vi "CRYAna Time.vi"(0 "Time Option":bool[](array[boolean]), 1 "Graph Info":T7={"Fs"=44100.0, "Channel Name"="Left", "Make Fundamental curve?"=FALSE}, 2 "TSR Info":T6 {"Impulse Resp Y" format="%.2f"; "Impulse Resp X" format="%.2f"}, 3 "Additive Info":T3, 5 "Stimulus":dbl[](array[numeric]), 7 "Input Info":T9, 9 "Response":dbl[](array[numeric]), 11 "Unit Info":T4={"Y unit In"="dB", "dB ref In"=1.0, "Y unit Out"="dB", "dB ref Out"=1.0, "Y unit Curve"="dB", "dB ref Curve"=1.0, "Y data  Curve"=0, "Y data Time"=0}, 12 "Algorithm":u16, 13 "Result Waveform":T8, 14 "EQ information":T2={"Stimulus EQ Curve"={"Name"="", "Curve"=[], "X data"=1, "Y data"=1, "Z data"=1, "X axis"=0, "Y axis"=1, "Z axis"=1, "X unit"="Hz", "Y unit"="", "Z unit"="deg.", "X dB ref"=1.0, "Y dB ref"=1.0, "Z dB ref"=1.0, "single val"=FALSE, "protected"=FALSE, "display X"=TRUE, "display Y"=TRUE, "display Z"=TRUE, "Test Info"="", "Step No."=0, "Plot Settings"={"Color"=0, "Interpolation"=0, "Point Style"=0, "Line Style"=0, "Point Color"=0, "Line Width"=0, "Bar Plot Style"=0, "Fill To"=0}, "AutoProtect"=FALSE}, "EQ"=FALSE, "EQ Rate"=0.0} {"EQ Rate" format="%.2f"; "Stimulus EQ Curve"."Z data" items=["dB", "Lin"]; "Stimulus EQ Curve"."X data" items=["dB", "Lin"]; "Stimulus EQ Curve"."Y data" items=["dB", "Lin"]; "Stimulus EQ Curve"."Z dB ref" format="%.1f"; "Stimulus EQ Curve"."Z axis" items=["Log", "Lin"]; "Stimulus EQ Curve"."X dB ref" format="%.1f"; "Stimulus EQ Curve"."X axis" items=["Log", "Lin"]; "Stimulus EQ Curve"."Y axis" items=["Log", "Lin"]; "Stimulus EQ Curve"."Y dB ref" format="%.1f"; "Stimulus EQ Curve"."Curve"."z" format="%.2f"; "Stimulus EQ Curve"."Curve"."y" format="%.2f"; "Stimulus EQ Curve"."Curve"."x" format="%.2f"}) -> (4 "Wave out":T5[](array[typedef]) {"Y dB ref" format="%.1f"; "Y axis" items=["Log", "Lin"]; "Y data" items=["dB", "Lin"]; "X data" items=["dB", "Lin"]})   [LabVIEW 2013]
uses:
  Typedef Control/CRYWaveform Cluster.ctl
  Typedef Control/CRYUnit Info Cluster.ctl
  Typedef Control/CRYData Cluster.ctl
  Typedef Control/CRYStimulus Test Infor Cluster.ctl
panel:
  in  "Waveform Cluster Out":T5={"Waveform"={"X0"=0.0, "dX"=0.0, "Y"=[]}, "X data"=1, "Y data"=0, "Y axis"=0, "X unit"="s", "Y unit"="", "Y dB ref"=1.0, "display Y"=TRUE, "display X"=FALSE, "Overload?"=FALSE, "Test Info"="", "Step No."=0, "Name"="", "protected"=FALSE, "Sqc history"=[], "Signal Channel ID"=0, "Plot Settings"={"Color"=0, "Interpolation"=0, "Point Style"=0, "Line Style"=0, "Point Color"=0, "Line Width"=0, "Bar Plot Style"=0, "Fill To"=0}, "AutoProtect"=FALSE} {"Y dB ref" format="%.1f"; "Y axis" items=["Log", "Lin"]; "Y data" items=["dB", "Lin"]; "X data" items=["dB", "Lin"]}
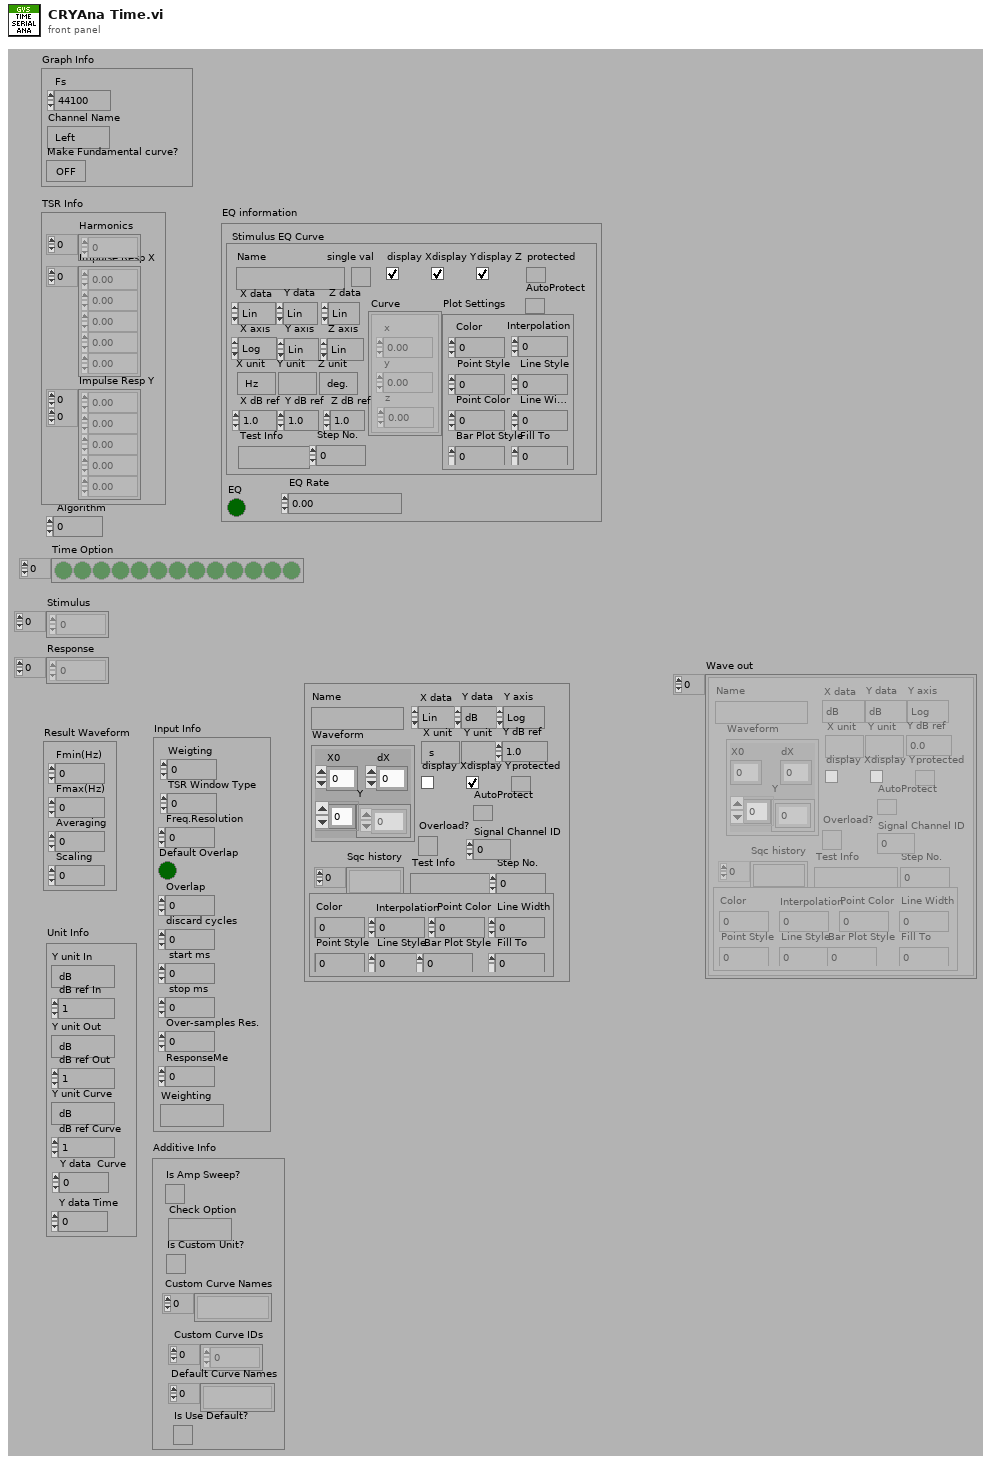
[diagram p1: front panel]
types:
  T1 = typedef "CRYData Cluster.ctl" = cluster{"Name":string, "Curve":cluster{"x":dbl, "y":dbl, "z":dbl}[], "X data":u16, "Y data":u16, "Z data":u16, "X axis":u16, "Y axis":u16, "Z axis":u16, "X unit":string, "Y unit":string, "Z unit":string, "X dB ref":dbl, "Y dB ref":dbl, "Z dB ref":dbl, "single val":bool, "protected":bool, "display X":bool, "display Y":bool, "display Z":bool, "Test Info":string, "Step No.":i32, "Plot Settings":cluster{"Color":u32, "Interpolation":u8, "Point Style":u8, "Line Style":u8, "Point Color":u32, "Line Width":u8, "Bar Plot Style":u8, "Fill To":i16}, "AutoProtect":bool}
  T2 = cluster{"Stimulus EQ Curve":T1, "EQ":bool, "EQ Rate":dbl}
  T3 = cluster{"Is Amp Sweep?":bool, "Check Option":string, "Is Custom Unit?":bool, "Custom Curve Names":string[], "Custom Curve IDs":i32[], "Default Curve Names":string[], "Is Use Default?":bool}
  T4 = typedef "CRYUnit Info Cluster.ctl" = cluster{"Y unit In":string, "dB ref In":dbl, "Y unit Out":string, "dB ref Out":dbl, "Y unit Curve":string, "dB ref Curve":dbl, "Y data  Curve":u16, "Y data Time":u16}
  T5 = typedef "CRYWaveform Cluster.ctl" = cluster{"Waveform":cluster{"X0":dbl, "dX":dbl, "Y":sgl[]}, "X data":u16, "Y data":u16, "Y axis":u16, "X unit":string, "Y unit":string, "Y dB ref":dbl, "display Y":bool, "display X":bool, "Overload?":bool, "Test Info":string, "Step No.":i32, "Name":string, "protected":bool, "Sqc history":string[], "Signal Channel ID":i32, "Plot Settings":cluster{"Color":u32, "Interpolation":u8, "Point Style":u8, "Line Style":u8, "Point Color":u32, "Line Width":u8, "Bar Plot Style":u8, "Fill To":i16}, "AutoProtect":bool}
  T6 = cluster{"Harmonics":dbl[], "Impulse Resp X":dbl[], "Impulse Resp Y":dbl[][]}
  T7 = cluster{"Fs":dbl, "Channel Name":string, "Make Fundamental curve?":bool}
  T8 = cluster{"Fmin(Hz)":dbl, "Fmax(Hz)":dbl, "Averaging":u16, "Scaling":u16}
  T9 = cluster{"Weigting":u16, "TSR Window Type":u16, "Freq.Resolution":dbl, "Default Overlap ":bool, "Overlap":dbl, "discard cycles":dbl, " start ms":dbl, " stop ms":dbl, "Over-samples Res.":dbl, "ResponseMe":u16, "Weighting":string}
  T10 = typedef "CRYStimulus Test Infor Cluster.ctl" = cluster{"Stimulus Type":string, "Signal Type":string, "In/Out":bool, "FAPS":cluster{"freq":dbl, "ampl":dbl, "cycles":dbl, "samples":i32}[], "Sampling Rate":dbl, "Samples":i32, "Analysis Param":string, "Resolution":u16, "Steps":u32, "Analysis Value":dbl[], "Diff Freq":dbl, "FStart":dbl, "FStop":dbl, "Calibration Param":string, "Anti Alias":dbl, "Level Out1":dbl, "Level Out2":dbl, "EQ":bool}
  T11 = cluster{"display X":bool, "display Y":bool, "display Z":bool}[]
  T12 = typedef "CRYUnit Info Out Cluster.ctl" = cluster{"X unit":string, "X data":u16, "Y unit":string, "Y data Time":u16, "Z unit":string, "X axis":u16, "X dB ref":dbl, "Y dB ref":dbl, "single/curve":bool}
  T13 = typedef "CRYAnalysis CurveName Cluster.ctl" = cluster{"Custom Curve Name":string, "Custom Curve ID":i32, "Default Curve Name":string}[]
  T14 = cluster{"Fs":dbl, "Freq.Resolution":dbl, "Overlap":dbl, "Weigting":u16}
  T15 = cluster{"display X":bool, "display Y":bool, "display Z":bool}
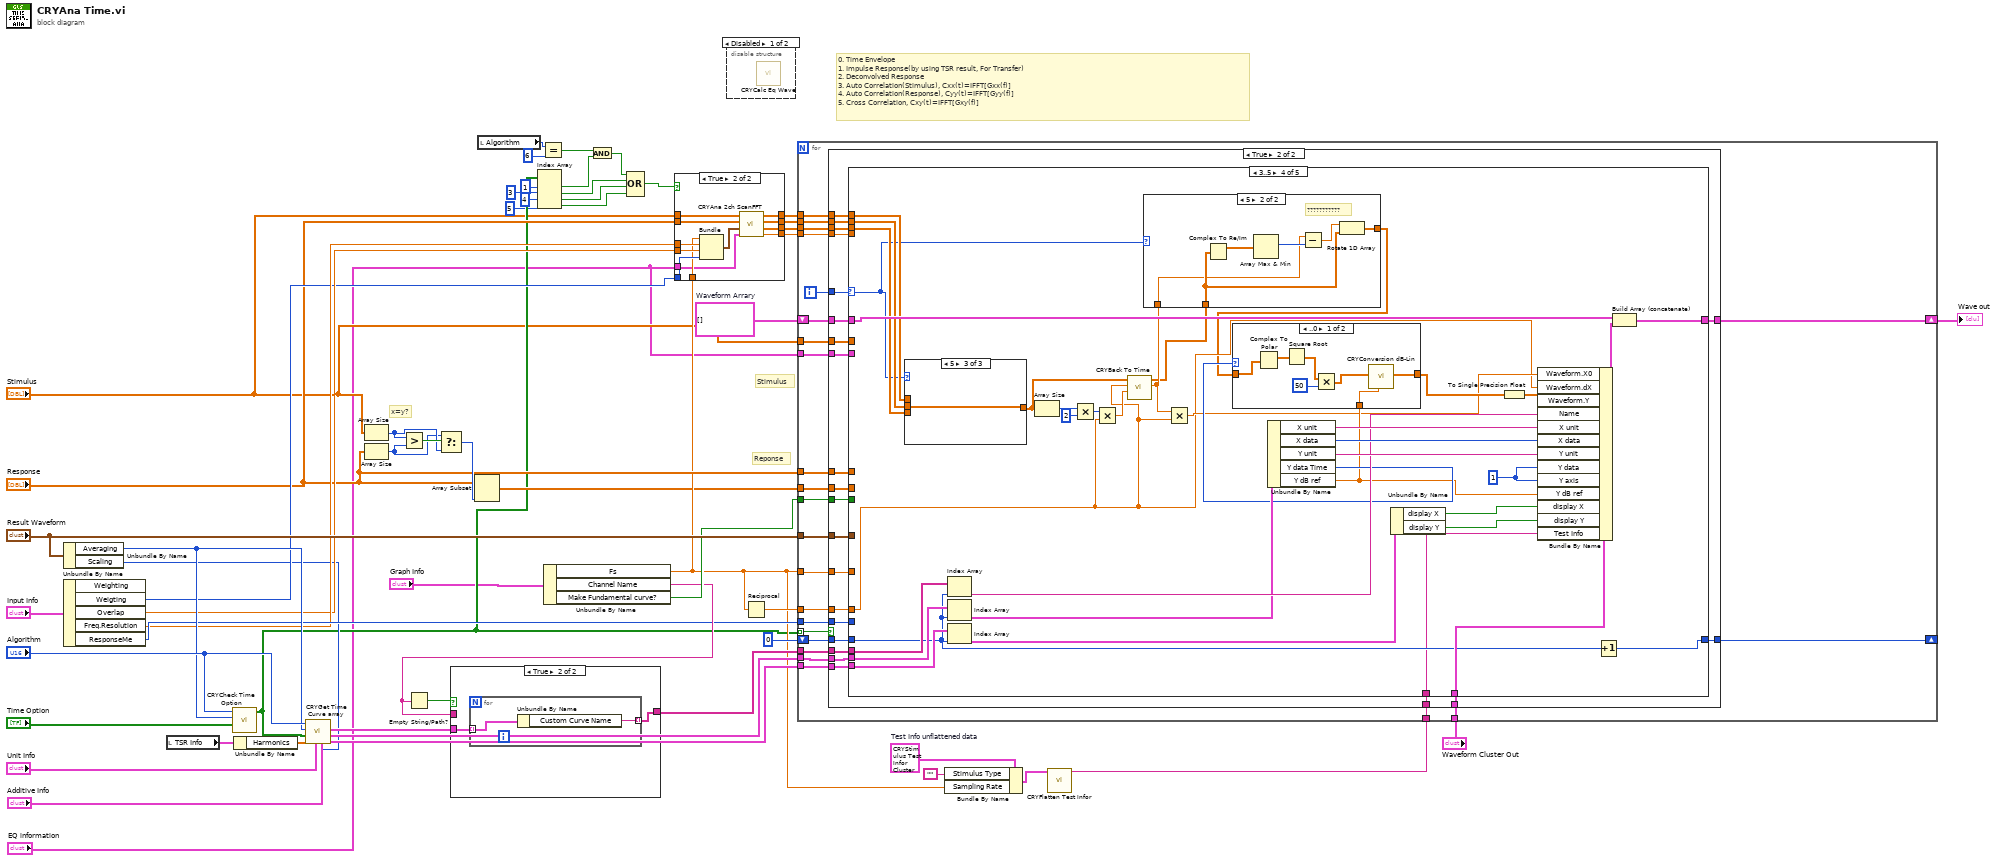
[diagram p0: block diagram]
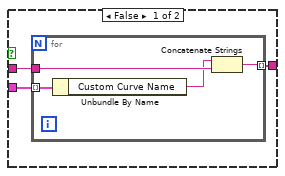
[diagram p4: hidden frame]
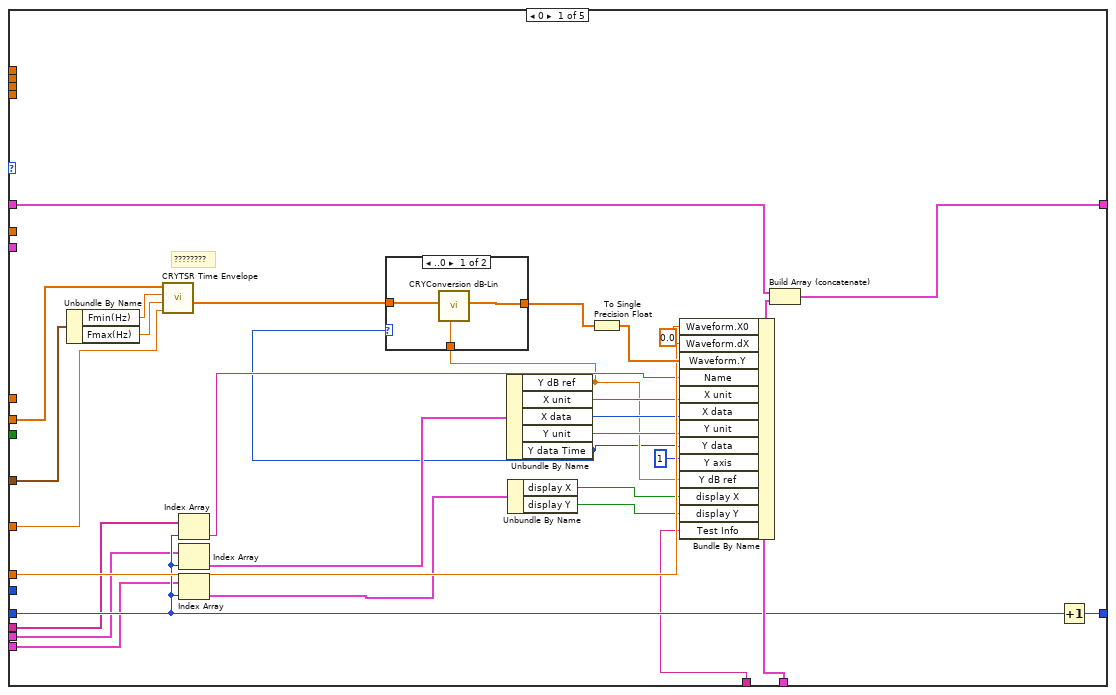
[diagram p6: hidden frame]
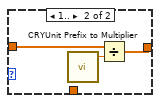
[diagram p7: hidden frame]
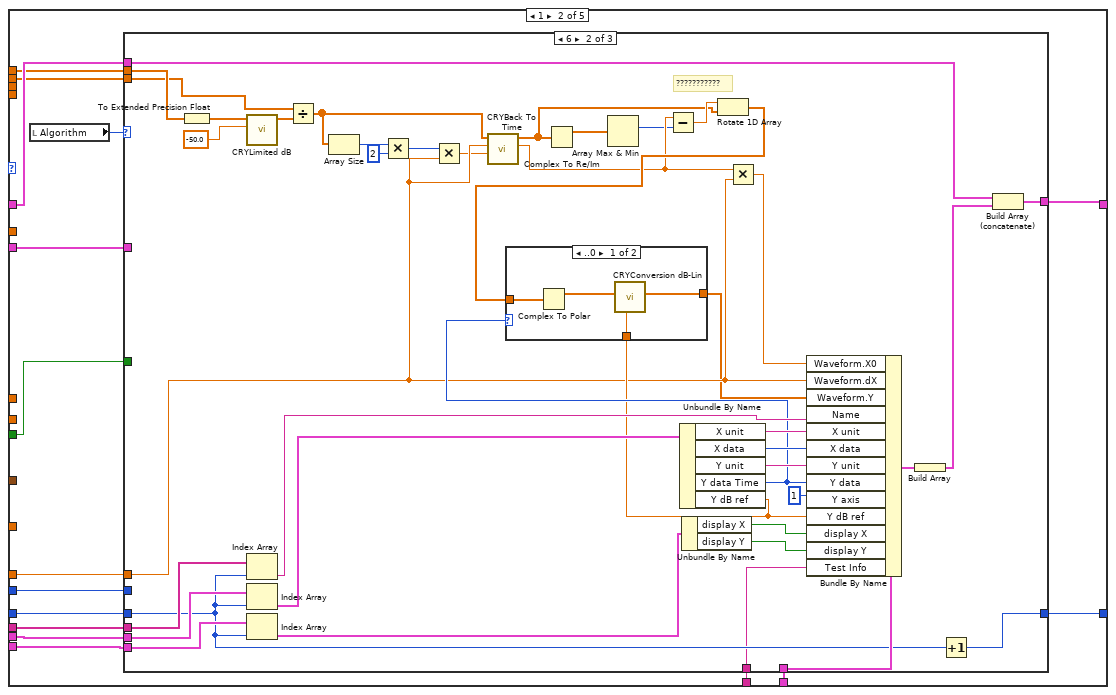
[diagram p8: hidden frame]
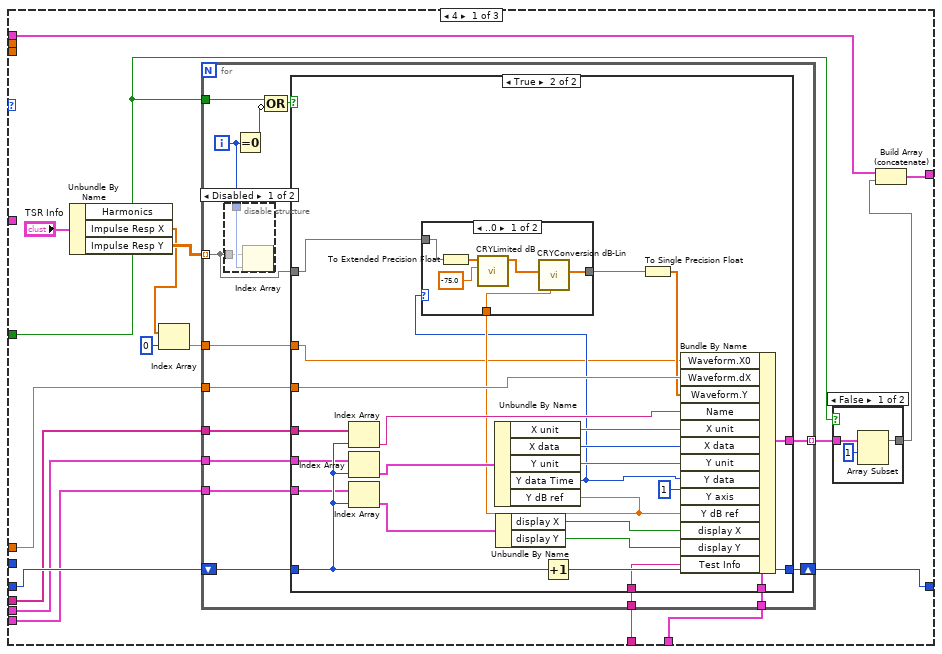
[diagram p9: hidden frame]
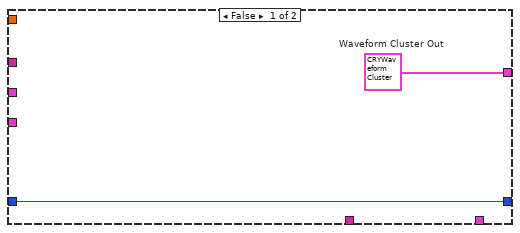
[diagram p12: hidden frame]
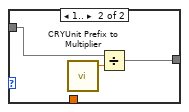
[diagram p13: hidden frame]
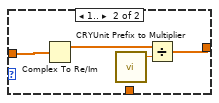
[diagram p14: hidden frame]
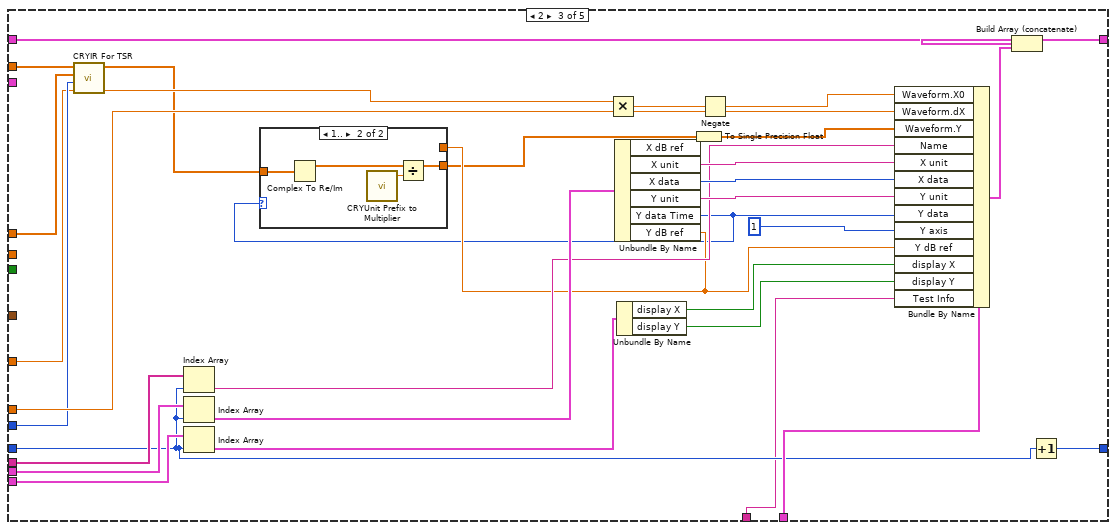
[diagram p16: hidden frame]
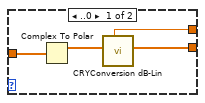
[diagram p17: hidden frame]
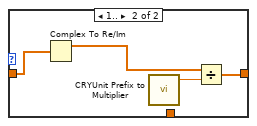
[diagram p19: hidden frame]
diagram:
  w23 = T10 {"Stimulus Type"="", "Signal Type"="", "In/Out"=FALSE, "FAPS"=[], "Sampling Rate"=0.0, "Samples"=0, "Analysis Param"="", "Resolution"=0, "Steps"=0, "Analysis Value"=[], "Diff Freq"=0.0, "FStart"=0.0, "FStop"=0.0, "Calibration Param"="", "Anti Alias"=0.0, "Level Out1"=0.0, "Level Out2"=0.0, "EQ"=FALSE}  # Test Info unflattened data
  w51 = T5[] []  # Waveform Arrary
  # "Reponse"
  # "0. Time Envelope\n1. Impulse Response(by using TSR result, For Transfer)\n2. Deconvolved Response\n3. Auto Correlation(Stimulus), Cxx(t)=IFFT[Gxx(f)]\n4. Auto Correlation(Response), Cyy(t)=IFFT[Gyy(f)]\n5. Cross Correlation, Cxy(t)=IFFT[Gxy(f)]"
  # "Stimulus"
  # "x=y?"
  n1 = Unbundle By Name("Result Waveform") -> ("Averaging"=w47:u16, "Scaling"=w26:u16)
  n2 = Unbundle By Name("Input Info") -> ("Weigting"=w28:u16, "Overlap"=w32:dbl, "Freq.Resolution"=w33:dbl, "ResponseMe"=w37:u16)  [unwired: 1 out]
  n3 = local read "TSR Info"() -> (w46:T6)
  n4 = call "CRYCheck Time Option.vi"("Option Array In"="Time Option", "Averaging"=w47, "Algorithm"="Algorithm") -> ("Option Array Out"=w18:bool[])  [unwired: 8 in]
  n5 = Unbundle By Name(w46) -> ("Harmonics"=w45:dbl[])
  n6 = call "CRYGet Time Curve array.vi"("Scaling"=w26, "Unit Info In"="Unit Info", "Additive Info"="Additive Info", "Harmonics array"=w45, "Option Array In"=w18, "Averaging"=w47, "Algorithm"="Algorithm") -> ("Display Array"=w43:T11, "Unit Info Out"=w44:T12[], "Curve Info Array Out"=w38:T13)  [unwired: 2 in]
  n7 = Array Size(array="Stimulus") -> (size(s)=w56:i32)
  n8 = Array Size(array="Response") -> (size(s)=w55:i32)
  n9 = Greater?(x=w56, y=w55) -> (0:w58:bool)
  n10 = Select(t=w55, s=w58, f=w56) -> (s? t:f=w57:i32)
  n11 = Array Subset(array="Response", length=w57) -> (w20:dbl[])  [unwired: 1 in]
  n12 = local read "Algorithm"() -> (w16:u16)
  n13 = Index Array(array=w18, index #1=1 ("index"), index #2=3 ("index"), index #3=4 ("index"), index #4=5 ("index")) -> (element #1=w13:bool, element #2=w8:bool, element #3=w7:bool, element #4=w6:bool)
  n14 = Equal?(x=w16, y=u16 6) -> (x = y?=w14:bool)
  n15 = Unbundle By Name("Graph Info") -> ("Fs"=w22:dbl, "Channel Name"=w40:string, "Make Fundamental curve?"=w50:bool)
  n16 = Empty String/Path?(string/path=w40) -> (empty?=w41:bool)
  n17 = case shown="True" w41 {
    tunnel: w38 -> [w61 w67]
    tunnel: w40 -> [w60 _]
    tunnel: [w59 w66] -> w39
    frame False {
      n18 = for {
        tunnel: w61 -> [w63] mode=indexing
        tunnel: w60 -> [w65]
        tunnel: [w64] -> w59 mode=indexing
        n19 = Unbundle By Name(w63) -> ("Custom Curve Name"=w62:string)
        n20 = Concatenate Strings(w62, w65) -> (w64:string)
      }
    }
    frame True {
      n21 = for {
        tunnel: w67 -> [w69] mode=indexing
        tunnel: [w68] -> w66 mode=indexing
        n22 = Unbundle By Name(w69) -> ("Custom Curve Name"=w68:string)
      }
    }
  }
  n23 = And(x=w14, y=w13) -> (x .and. y?=w9:bool)
  n24 = Compound Arithmetic op=OR(w9, w8, w7, w6) -> (w5:bool)
  n25 = case shown="True" w5 {
    tunnel: [_ w81] -> w35
    tunnel: [_ w80] -> w34
    tunnel: w33 -> [_ w79]
    tunnel: w32 -> [_ w78]
    tunnel: [_ w76] -> w30
    tunnel: [_ w75] -> w29
    tunnel: w28 -> [_ w74]
    tunnel: "Response" -> [_ w73]
    tunnel: w22 -> [_ w72]
    tunnel: "Stimulus" -> [_ w71]
    tunnel: "EQ information" -> [_ w70]
    frame False {
    }
    frame True {
      n26 = Bundle("Fs"=w72, "Freq.Resolution"=w79, "Overlap"=w78, "Weigting"=w74) -> (w77:T14)  [unwired: 1 in]
      n27 = call "CRYAna 2ch ScanFFT.vi"("EQ information"=w70, "In Parameter"=w77, "Response[y(t)]"=w73, "Stimulus[x(t)]"=w71) -> ("New dF(Hz)"=w80:dbl, "Gyy"=w81:dbl[], "Gxy"=w75:cdb[], "Gxx"=w76:dbl[])  [unwired: 4 in]
    }
  }
  n28 = disable-structure shown="Disabled" {
    frame Disabled {
      n29 = call "CRYCalc Eq Wave.vi"() -> ()  [unwired: 10 in, 2 out]
    }
    frame Enabled {
    }
  }
  n30 = Reciprocal(x=w22) -> (1/x=w31:dbl)
  n31 = Bundle By Name(cluster=w23, "Stimulus Type"="", "Sampling Rate"=w22) -> (w24:T10)
  n32 = call "CRYFlatten Test Infor.vi"("Test Infor data"=w24) -> ("Fattened Data"=w21:string)  [unwired: 10 out]
  n33 = for {
    tunnel: w18 -> [w104] mode=indexing
    tunnel: w31 -> [w103]
    tunnel: "Result Waveform" -> [w98]
    tunnel: "Waveform Cluster Out" -> [w102]
    shift-right: [w101] -> w19
    shift-left: w51 -> [w100]
    tunnel: w22 -> [w99]
    tunnel: w50 -> [w97]
    tunnel: w39 -> [w94]
    tunnel: w44 -> [w93]
    tunnel: w43 -> [w92]
    shift-right: [w96] -> _
    shift-left: 0 -> [w95]
    tunnel: w20 -> [w91]
    tunnel: "Stimulus" -> [w90]
    tunnel: "Response" -> [w89]
    tunnel: w37 -> [w88]
    tunnel: w30 -> [w87]
    tunnel: w29 -> [w86]
    tunnel: w35 -> [w85]
    tunnel: w34 -> [w84]
    tunnel: w21 -> [w83]
    tunnel: "EQ information" -> [w82]
    i -> [w105]
    n34 = case shown="True" w104 {
      tunnel: w105 -> [_ w130]
      tunnel: w103 -> [_ w129]
      tunnel: w102 -> [_ w128]
      tunnel: [w107 w127] -> w101
      tunnel: w100 -> [w107 w126]
      tunnel: w99 -> [_ w125]
      tunnel: w98 -> [_ w124]
      tunnel: w97 -> [_ w123]
      tunnel: w95 -> [w106 w122]
      tunnel: [w106 w121] -> w96
      tunnel: w94 -> [_ w120]
      tunnel: w93 -> [_ w119]
      tunnel: w92 -> [_ w118]
      tunnel: w91 -> [_ w117]
      tunnel: w90 -> [_ w116]
      tunnel: w89 -> [_ w115]
      tunnel: w88 -> [_ w114]
      tunnel: w87 -> [_ w113]
      tunnel: w86 -> [_ w112]
      tunnel: w85 -> [_ w111]
      tunnel: w84 -> [_ w110]
      tunnel: w83 -> [_ w109]
      tunnel: w82 -> [_ w108]
      frame False {
      }
      frame True {
        n35 = case shown="3..5" w130 {
          selector: w130 -> [_ _ _ w354 _]
          tunnel: w129 -> [w152 w182 w335 w355 _]
          tunnel: w128 -> [w158 w183 w337 w382 _]
          tunnel: [w156 w173 w338 w384 w408] -> w127
          tunnel: w126 -> [w155 w174 w336 w385 w408]
          tunnel: w125 -> [w132 _ w310 _ _]
          tunnel: w124 -> [w154 _ _ _ _]
          tunnel: w123 -> [_ w181 _ _ _]
          tunnel: w122 -> [w144 w176 w320 w372 w407]
          tunnel: [w145 w175 w319 w371 w407] -> w121
          tunnel: w120 -> [w143 w179 w326 w375 _]
          tunnel: w119 -> [w142 w178 w325 w374 _]
          tunnel: w118 -> [w141 w177 w324 w373 _]
          tunnel: w117 -> [w137 _ _ _ _]
          tunnel: w116 -> [_ _ w315 _ _]
          tunnel: w115 -> [_ _ w314 _ _]
          tunnel: w114 -> [_ w172 w312 _ _]
          tunnel: w113 -> [_ w171 _ w363 _]
          tunnel: w112 -> [_ w170 _ w364 _]
          tunnel: w111 -> [_ _ _ w365 _]
          tunnel: w110 -> [_ _ _ _ _]
          tunnel: w109 -> [w131 w169 w309 w349 _]
          tunnel: w108 -> [_ w168 _ _ _]
          frame 0 {
            # "????????"
            n36 = Unbundle By Name(w154) -> ("Fmin(Hz)"=w160:dbl, "Fmax(Hz)"=w161:dbl)
            n37 = call "CRYTSR Time Envelope.vi"("Fs"=w132, "FMax"=w161, "FMin"=w160, "Response"=w137) -> ("Magn"=w133:dbl[])  [unwired: 5 in, 2 out]
            n38 = Index Array(array=w143, index=w144) -> (element=w140:string)
            n39 = Index Array(array=w142, index=w144) -> (element=w139:T12)
            n40 = Index Array(array=w141, index=w144) -> (element=w138:T15)
            n41 = Unbundle By Name(w139) -> ("Y dB ref"=w135:dbl, "X unit"=w148:string, "X data"=w147:u16, "Y unit"=w149:string, "Y data Time"=w134:u16)
            n42 = case shown="..0" w134 {
              tunnel: w133 -> [w163 w167]
              tunnel: w135 -> [w164 _]
              tunnel: [w162 w165] -> w136
              frame ..0 {
                n43 = call "CRYConversion dB-Lin.vi"("dB ref."=w164, "Lin In array"=w163) -> ("Log Out array"=w162:dbl[])  [unwired: 4 in, 3 out]
              }
              frame 1.. {
                n44 = call "CRYUnit Prefix to Multiplier.vi"() -> ("multiplier"=w166:dbl)  [unwired: 1 in, 4 out]
                n45 = Divide(x=w167, y=w166) -> (x/y=w165:dbl[])
              }
            }
            n46 = Unbundle By Name(w138) -> ("display X"=w151:bool, "display Y"=w150:bool)
            n47 = To Single Precision Float(number=w136) -> (single precision float=w153:sgl[])
            n48 = Bundle By Name(cluster=w158, "Waveform.X0"=0.0, "Waveform.dX"=w152, "Waveform.Y"=w153, "Name"=w140, "X unit"=w148, "X data"=w147, "Y unit"=w149, "Y data"=w134, "Y axis"=u16 1, "Y dB ref"=w135, "display X"=w151, "display Y"=w150, "Test Info"=w131) -> (w157:T5)
            n49 = Build Array (concatenate)(w155, w157) -> (w156:T5[])
            n50 = Increment(x=w144) -> (x+1=w145:i32)
          }
          frame 1 {
            n51 = local read "Algorithm"() -> (w180:u16)
            n52 = case shown="6" w180 {
              tunnel: w183 -> [w200 w298 _]
              tunnel: w182 -> [w199 w271 _]
              tunnel: w181 -> [w198 _ _]
              tunnel: w179 -> [w191 w291 _]
              tunnel: w178 -> [w189 w290 _]
              tunnel: w177 -> [w188 w289 _]
              tunnel: w176 -> [w192 w288 w308]
              tunnel: [w190 w287 w308] -> w175
              tunnel: w174 -> [w195 w283 w307]
              tunnel: [w193 w281 w307] -> w173
              tunnel: w172 -> [_ _ _]
              tunnel: w171 -> [_ w268 _]
              tunnel: w170 -> [_ w267 _]
              tunnel: w169 -> [w187 w258 _]
              tunnel: w168 -> [_ _ _]
              frame 4 {
                n53 = Unbundle By Name("TSR Info") -> ("Impulse Resp X"=w185:dbl[], "Impulse Resp Y"=w196:dbl[][])  [unwired: 1 out]
                n54 = Index Array(array=w185, index=0) -> (element=w184:dbl)
                n55 = for {
                  tunnel: [w220] -> w201 mode=indexing
                  tunnel: w196 -> [w206] mode=indexing
                  tunnel: w198 -> [w218]
                  tunnel: w200 -> [w216]
                  tunnel: w199 -> [w215]
                  tunnel: w191 -> [w213]
                  tunnel: w189 -> [w211]
                  tunnel: w188 -> [w210]
                  shift-right: [w212] -> w190
                  shift-left: w192 -> [w214]
                  tunnel: w187 -> [w208]
                  tunnel: w184 -> [w207]
                  i -> [w209]
                  n56 = disable-structure shown="Disabled" {
                    disable-tunnel: w209 -> [w222 _]
                    disable-tunnel: w206 -> [w221 _]
                    frame Disabled {
                      n57 = Index Array(array=w221, index=w222) -> ()  [unwired: 1 out]
                    }
                    frame Enabled {
                    }
                  }
                  n58 = Equal To 0?(x=w209) -> (x = 0?=w219:bool)
                  n59 = Compound Arithmetic op=OR(w218, invert w219) -> (w217:bool)
                  n60 = case shown="True" w217 {
                    tunnel: [w224 w247] -> w220
                    tunnel: w206 -> [_ w227]
                    tunnel: w216 -> [_ w248]
                    tunnel: w215 -> [_ w246]
                    tunnel: w214 -> [w223 w238]
                    tunnel: w213 -> [_ w239]
                    tunnel: [w223 w237] -> w212
                    tunnel: w211 -> [_ w236]
                    tunnel: w210 -> [_ w235]
                    tunnel: w208 -> [_ w226]
                    tunnel: w207 -> [_ w225]
                    frame False {
                      w224 = T5 {"Waveform"={"X0"=0.0, "dX"=0.0, "Y"=[]}, "X data"=1, "Y data"=1, "Y axis"=1, "X unit"="s", "Y unit"="V", "Y dB ref"=1.0, "display Y"=TRUE, "display X"=TRUE, "Overload?"=FALSE, "Test Info"="", "Step No."=0, "Name"="", "protected"=FALSE, "Sqc history"=[], "Signal Channel ID"=0, "Plot Settings"={"Color"=0, "Interpolation"=0, "Point Style"=0, "Line Style"=0, "Point Color"=0, "Line Width"=0, "Bar Plot Style"=0, "Fill To"=0}, "AutoProtect"=FALSE}  # Waveform Cluster Out
                    }
                    frame True {
                      n61 = Index Array(array=w239, index=w238) -> (element=w234:string)
                      n62 = Index Array(array=w236, index=w238) -> (element=w233:T12)
                      n63 = Index Array(array=w235, index=w238) -> (element=w232:T15)
                      n64 = Unbundle By Name(w233) -> ("X unit"=w243:string, "X data"=w242:u16, "Y unit"=w241:string, "Y data Time"=w228:u16, "Y dB ref"=w229:dbl)
                      n65 = case shown="..0" w228 {
                        tunnel: w227 -> [w250 w257]
                        tunnel: w229 -> [w254 _]
                        tunnel: [w253 w255] -> w230
                        frame ..0 {
                          n66 = To Extended Precision Float(1:w250) -> (0:w252:ext[])
                          n67 = call "CRYLimited dB.vi"("Dynamic(dB)"=-75.0, "Power spectrum"=w252) -> ("Limited spectrum"=w249:ext[])  [unwired: 9 in]
                          n68 = call "CRYConversion dB-Lin.vi"("dB ref."=w254, "Lin In array"=w249) -> ("Log Out array"=w253:dbl[])  [unwired: 4 in, 3 out]
                        }
                        frame 1.. {
                          n69 = call "CRYUnit Prefix to Multiplier.vi"() -> ("multiplier"=w256:dbl)  [unwired: 1 in, 4 out]
                          n70 = Divide(x=w257, y=w256) -> (x/y=w255:dbl[])
                        }
                      }
                      n71 = Unbundle By Name(w232) -> ("display X"=w245:bool, "display Y"=w244:bool)
                      n72 = Increment(x=w238) -> (x+1=w237:i32)
                      n73 = To Single Precision Float(number=w230) -> (single precision float=w231:sgl[])
                      n74 = Bundle By Name(cluster=w248, "Waveform.X0"=w225, "Waveform.dX"=w246, "Waveform.Y"=w231, "Name"=w234, "X unit"=w243, "X data"=w242, "Y unit"=w241, "Y data"=w228, "Y axis"=u16 1 ("X data"), "Y dB ref"=w229, "display X"=w245, "display Y"=w244, "Test Info"=w226) -> (w247:T5)
                    }
                  }
                }
                n75 = case shown="False" w198 {
                  tunnel: [w202 w205] -> w194
                  tunnel: w201 -> [w203 w205]
                  frame False {
                    n76 = Array Subset(array=w203, index=1 ("Array Index")) -> (w202:T5[])  [unwired: 1 in]
                  }
                  frame True {
                  }
                }
                n77 = Build Array (concatenate)(w195, w194) -> (w193:T5[])
              }
              frame 6 {
                # "???????????"
                n78 = To Extended Precision Float(1:w268) -> (0:w277:ext[])
                n79 = call "CRYLimited dB.vi"("Dynamic(dB)"=-50.0, "Power spectrum"=w277) -> ("Limited spectrum"=w275:ext[])  [unwired: 9 in]
                n80 = Index Array(array=w291, index=w288) -> (element=w286:string)
                n81 = Index Array(array=w290, index=w288) -> (element=w285:T12)
                n82 = Index Array(array=w289, index=w288) -> (element=w284:T15)
                n83 = Divide(x=w267, y=w275) -> (x/y=w269:cxt[])
                n84 = Array Size(array=w269) -> (size(s)=w274:i32)
                n85 = Multiply(x=w274, y=2) -> (x*y=w272:i32)
                n86 = Multiply(x=w272, y=w271) -> (x*y=w270:dbl)
                n87 = call "CRYBack To Time.vi"("T(s)"=w270, "dt(s)"=w271, "Spectrum"=w269) -> ("t0S"=w261:dbl, "timeHistory"=w259:cdb[])  [unwired: 7 in]
                n88 = Complex To Re/Im(x + iy=w259) -> (x=w266:dbl[])  [unwired: 1 out]
                n89 = Array Max & Min(array=w266) -> (max index (indices)=w260:i32)  [unwired: 3 out]
                n90 = Subtract(x=w261, y=w260) -> (x-y=w264:dbl)
                n91 = Unbundle By Name(w285) -> ("X unit"=w295:string, "X data"=w294:u16, "Y unit"=w293:string, "Y data Time"=w280:u16, "Y dB ref"=w279:dbl)
                n92 = Unbundle By Name(w284) -> ("display X"=w297:bool, "display Y"=w296:bool)
                n93 = Rotate 1D Array(1:w259, 2:w264) -> (0:w265:cdb[])
                n94 = case shown="..0" w280 {
                  tunnel: w265 -> [w300 w304]
                  tunnel: w279 -> [w302 _]
                  tunnel: [w301 w305] -> w262
                  frame ..0 {
                    n95 = Complex To Polar(r * e^(i*theta)=w300) -> (r=w299:dbl[])  [unwired: 1 out]
                    n96 = call "CRYConversion dB-Lin.vi"("dB ref."=w302, "Lin In array"=w299) -> ("Log Out array"=w301:dbl[])  [unwired: 4 in, 3 out]
                  }
                  frame 1.. {
                    n97 = Complex To Re/Im(x + iy=w304) -> (x=w303:dbl[])  [unwired: 1 out]
                    n98 = call "CRYUnit Prefix to Multiplier.vi"() -> ("multiplier"=w306:dbl)  [unwired: 1 in, 4 out]
                    n99 = Divide(x=w303, y=w306) -> (x/y=w305:dbl[])
                  }
                }
                n100 = Multiply(x=w261, y=w271) -> (x*y=w276:dbl)
                n101 = Bundle By Name(cluster=w298, "Waveform.X0"=w276, "Waveform.dX"=w271, "Waveform.Y"=w262, "Name"=w286, "X unit"=w295, "X data"=w294, "Y unit"=w293, "Y data"=w280, "Y axis"=u16 1, "Y dB ref"=w279, "display X"=w297, "display Y"=w296, "Test Info"=w258) -> (w263:T5)
                n102 = Build Array(w263) -> (w282:T5[])
                n103 = Increment(x=w288) -> (x+1=w287:i32)
                n104 = Build Array (concatenate)(w283, w282) -> (w281:T5[])
              }
              frame Default {
              }
            }
          }
          frame 2 {
            n105 = call "CRYIR For TSR.vi"("Fs"=w310, "Abs/Rel"=w312, "Response[y(t)]"=w314, "Stimulus[x(t)]"=w315) -> ("T0"=w313:dbl, "Deconvolved Response"=w311:cdb[])  [unwired: 3 in, 3 out]
            n106 = Index Array(array=w326, index=w320) -> (element=w321:string)
            n107 = Index Array(array=w325, index=w320) -> (element=w322:T12)
            n108 = Index Array(array=w324, index=w320) -> (element=w323:T15)
            n109 = Multiply(x=w313, y=w335) -> (x*y=w340:dbl)
            n110 = Unbundle By Name(w322) -> ("X unit"=w330:string, "X data"=w329:u16, "Y unit"=w328:string, "Y data Time"=w317:u16, "Y dB ref"=w318:dbl)  [unwired: 1 out]
            n111 = case shown="1.." w317 {
              tunnel: [w344 w347] -> w316
              tunnel: w318 -> [w343 _]
              tunnel: w311 -> [w342 w346]
              frame ..0 {
                n112 = Complex To Polar(r * e^(i*theta)=w342) -> (r=w341:dbl[])  [unwired: 1 out]
                n113 = call "CRYConversion dB-Lin.vi"("dB ref."=w343, "Lin In array"=w341) -> ("Log Out array"=w344:dbl[])  [unwired: 4 in, 3 out]
              }
              frame 1.. {
                n114 = Complex To Re/Im(x + iy=w346) -> (x=w345:dbl[])  [unwired: 1 out]
                n115 = call "CRYUnit Prefix to Multiplier.vi"() -> ("multiplier"=w348:dbl)  [unwired: 1 in, 4 out]
                n116 = Divide(x=w345, y=w348) -> (x/y=w347:dbl[])
              }
            }
            n117 = Unbundle By Name(w323) -> ("display X"=w333:bool, "display Y"=w332:bool)
            n118 = To Single Precision Float(number=w316) -> (single precision float=w327:sgl[])
            n119 = Negate(x=w340) -> (-x=w334:dbl)
            n120 = Bundle By Name(cluster=w337, "Waveform.X0"=w334, "Waveform.dX"=w335, "Waveform.Y"=w327, "Name"=w321, "X unit"=w330, "X data"=w329, "Y unit"=w328, "Y data"=w317, "Y axis"=u16 1, "Y dB ref"=w318, "display X"=w333, "display Y"=w332, "Test Info"=w309) -> (w339:T5)
            n121 = Build Array (concatenate)(w336, w339) -> (w338:T5[])
            n122 = Increment(x=w320) -> (x+1=w319:i32)
          }
          frame 3..5 {
            w351 = u16 1 ("Y axis")
            n123 = case shown="5" w354 {
              tunnel: w363 -> [w404 _ _]
              tunnel: w365 -> [_ w405 _]
              tunnel: [w404 w405 w406] -> w357
              tunnel: w364 -> [_ _ w406]
              frame 3, Default {
              }
              frame 4 {
              }
              frame 5 {
              }
            }
            n124 = Index Array(array=w375, index=w372) -> (element=w370:string)
            n125 = Index Array(array=w374, index=w372) -> (element=w369:T12)
            n126 = Index Array(array=w373, index=w372) -> (element=w368:T15)
            n127 = Array Size(array=w357) -> (size(s)=w361:i32)
            n128 = Multiply(x=w361, y=2) -> (x*y=w359:i32)
            n129 = Multiply(x=w359, y=w355) -> (x*y=w358:dbl)
            n130 = call "CRYBack To Time.vi"("T(s)"=w358, "dt(s)"=w355, "Spectrum"=w357) -> ("t0S"=w352:dbl, "timeHistory"=w350:cdb[])  [unwired: 7 in]
            n131 = case shown="5" w354 {
              tunnel: w350 -> [w386 w388]
              tunnel: [w386 w389] -> w353
              tunnel: w352 -> [_ w387]
              frame 0, Default {
              }
              frame 5 {
                # "???????????"
                n132 = Complex To Re/Im(x + iy=w388) -> (x=w392:dbl[])  [unwired: 1 out]
                n133 = Array Max & Min(array=w392) -> (max index (indices)=w390:i32)  [unwired: 3 out]
                n134 = Subtract(x=w387, y=w390) -> (x-y=w391:dbl)
                n135 = Rotate 1D Array(1:w388, 2:w391) -> (0:w389:cdb[])
              }
            }
            n136 = Multiply(x=w352, y=w355) -> (x*y=w356:dbl)
            n137 = Unbundle By Name(w369) -> ("X unit"=w378:string, "X data"=w376:u16, "Y unit"=w377:string, "Y data Time"=w367:u16, "Y dB ref"=w366:dbl)
            n138 = case shown="..0" w367 {
              tunnel: w353 -> [w396 w401]
              tunnel: w366 -> [w399 _]
              tunnel: [w398 w403] -> w362
              frame ..0 {
                n139 = Complex To Polar(r * e^(i*theta)=w396) -> (r=w394:dbl[])  [unwired: 1 out]
                n140 = Square Root(x=w394) -> (sqrt(x)=w393:dbl[])
                n141 = Multiply(x=w393, y=50) -> (x*y=w395:dbl[])
                n142 = call "CRYConversion dB-Lin.vi"("dB ref."=w399, "Lin In array"=w395) -> ("Log Out array"=w398:dbl[])  [unwired: 4 in, 3 out]
              }
              frame 1.. {
                n143 = Complex To Re/Im(x + iy=w401) -> (x=w400:dbl[])  [unwired: 1 out]
                n144 = call "CRYUnit Prefix to Multiplier.vi"() -> ("multiplier"=w402:dbl)  [unwired: 1 in, 4 out]
                n145 = Divide(x=w400, y=w402) -> (x/y=w403:dbl[])
              }
            }
            n146 = Unbundle By Name(w368) -> ("display X"=w380:bool, "display Y"=w379:bool)
            n147 = To Single Precision Float(number=w362) -> (single precision float=w381:sgl[])
            n148 = Bundle By Name(cluster=w382, "Waveform.X0"=w356, "Waveform.dX"=w355, "Waveform.Y"=w381, "Name"=w370, "X unit"=w378, "X data"=w376, "Y unit"=w377, "Y data"=w351, "Y axis"=w351, "Y dB ref"=w366, "display X"=w380, "display Y"=w379, "Test Info"=w349) -> (w383:T5)
            n149 = Increment(x=w372) -> (x+1=w371:i32)
            n150 = Build Array (concatenate)(w385, w383) -> (w384:T5[])
          }
          frame Default {
          }
        }
      }
    }
  }
  "Wave out" <- w19
